vi "The Shell.vi"() -> ()   [LabVIEW 2010]
uses:
  Global variables/Parameters.glb
panel:
  in  "Directory for Saved Data":path=path "D:/Data"
  out "found match":bool
  in  "New session?":bool
  in  "Animal type":u16(ring) items=["Frog", "Gecko", "Chicken", "Probe", "Lamprey"]
  in  "New ear?":bool
  out "Instructions":string="Click once on your name; then select OK.  "
  in  "Stop.":bool
  in  "New cell?":bool
  in  "OK.":bool
  out "Choice":string
  out "Display.":string
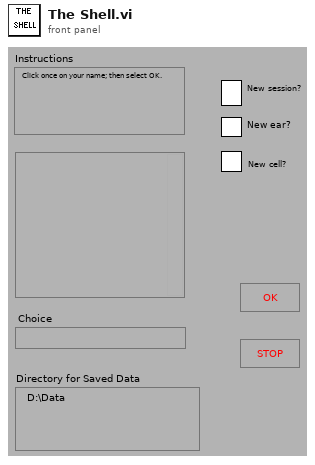
[diagram p1: front panel]
types:
  T1 = enum16{"open", "replace", "create", "open or create", "replace or create", "replace or create with confirmation"}
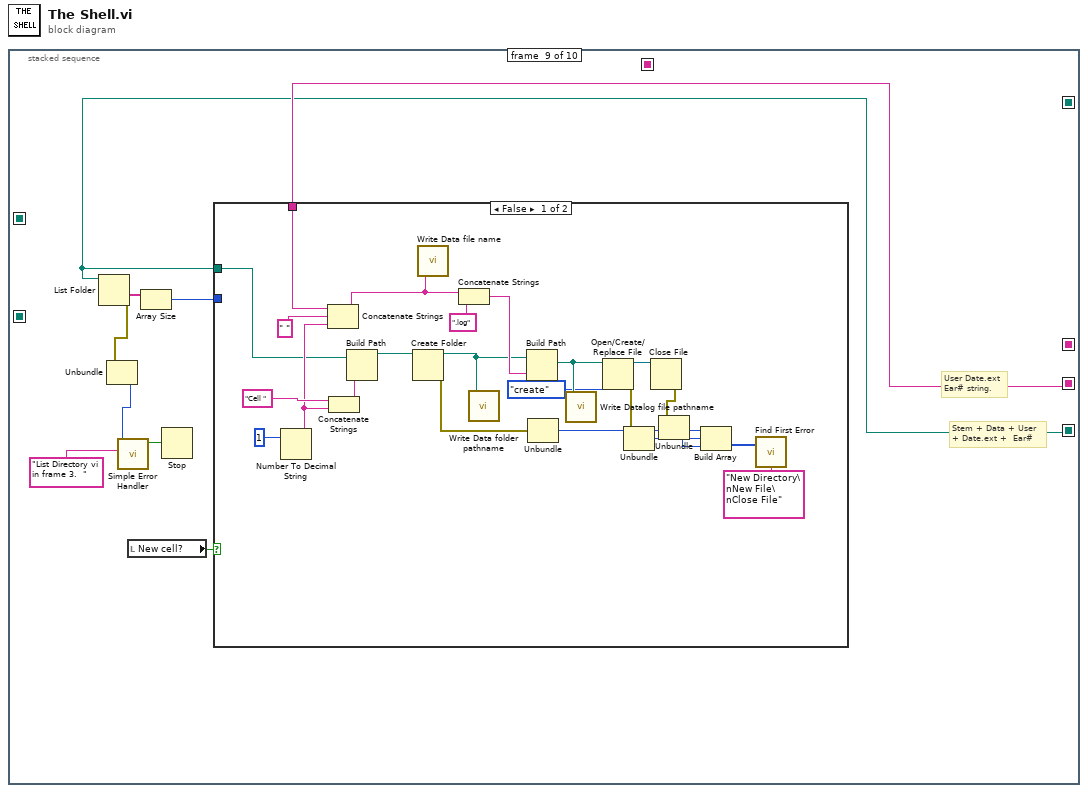
[diagram p0: block diagram]
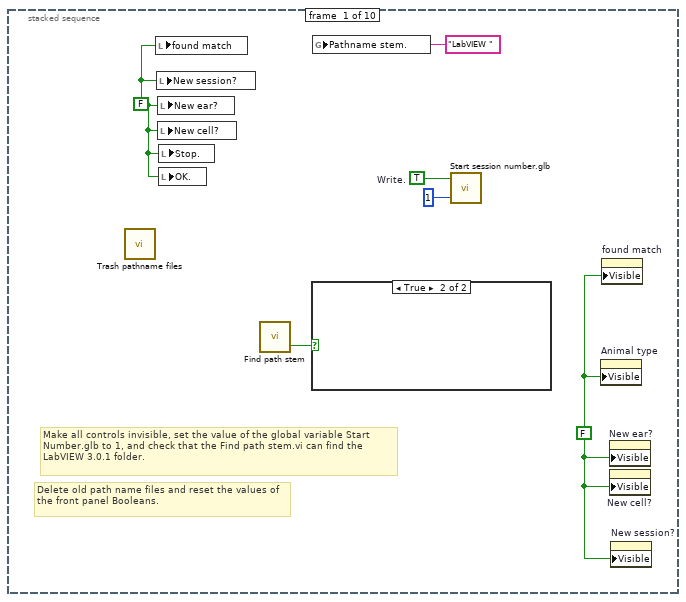
[diagram p2: hidden frame]
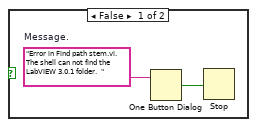
[diagram p3: hidden frame]
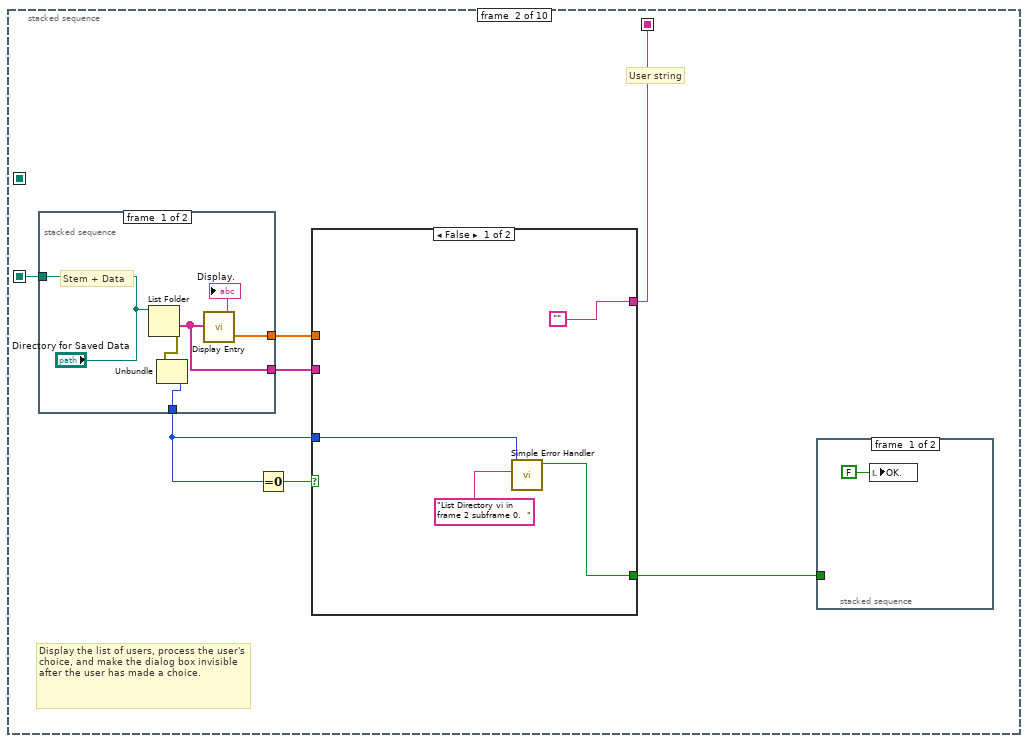
[diagram p4: hidden frame]
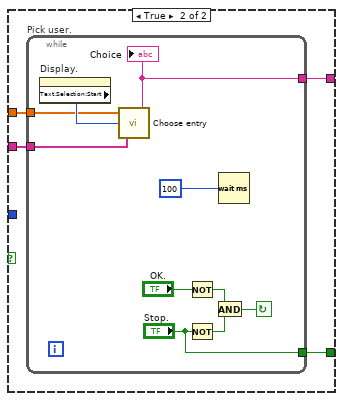
[diagram p5: hidden frame]
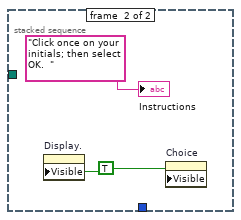
[diagram p6: hidden frame]
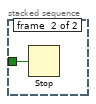
[diagram p7: hidden frame]
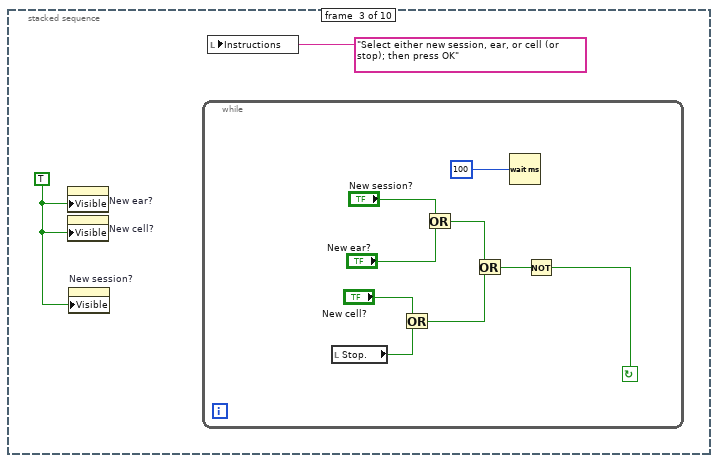
[diagram p8: hidden frame]
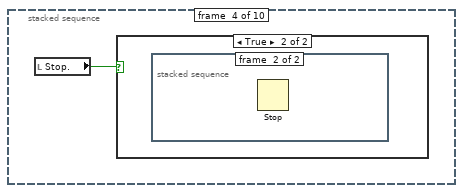
[diagram p9: hidden frame]
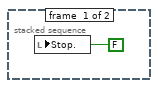
[diagram p11: hidden frame]
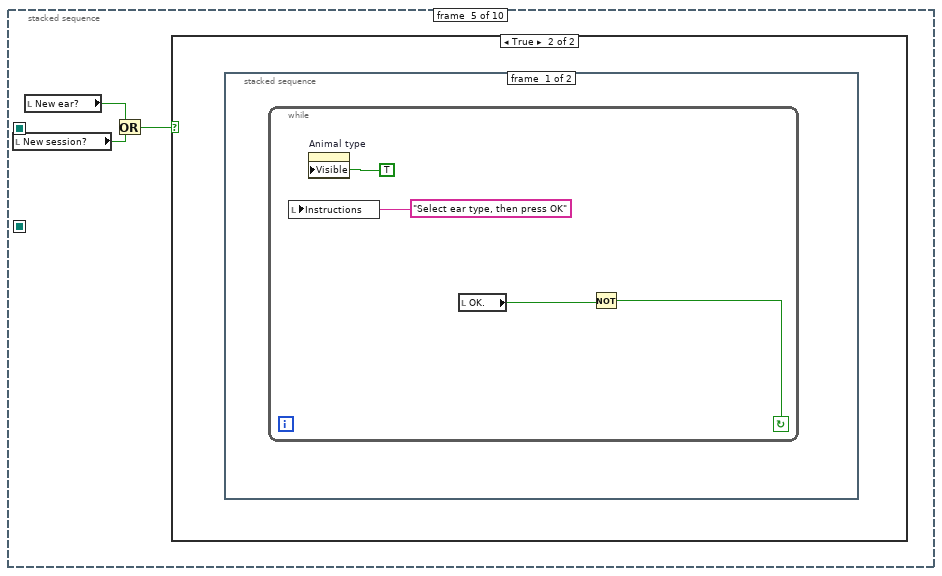
[diagram p12: hidden frame]
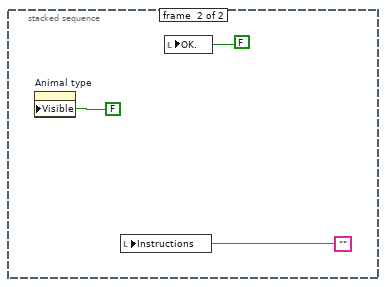
[diagram p14: hidden frame]
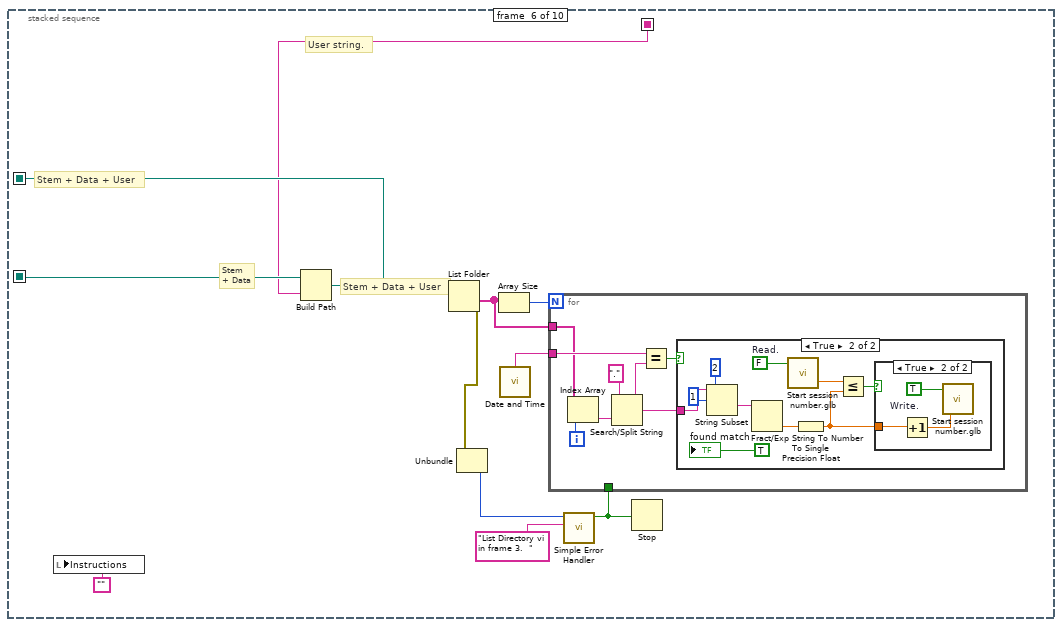
[diagram p15: hidden frame]
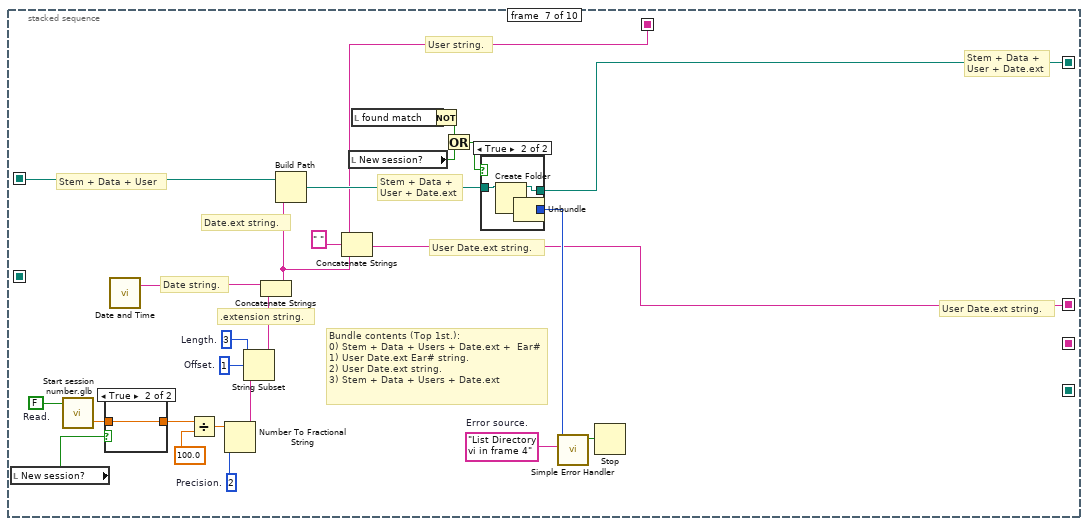
[diagram p18: hidden frame]
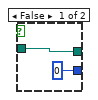
[diagram p19: hidden frame]
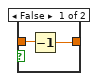
[diagram p20: hidden frame]
diagram:
  n1 = stacked-sequence {
    seq-local: [_ w10 _ _ _ _ _ _ _ _] -> [_ _ _ _ _ w68 w99 _ _ _]
    seq-local: [_ w15 _ _ _ _ _ _ _ _] -> [_ _ _ _ _ w76 _ _ _ _]
    seq-local: [_ _ _ _ _ w69 _ _ _ _] -> [_ _ _ _ _ _ w111 _ _ _]
    seq-local: [_ _ _ _ _ _ w105 _ _ _] -> [_ _ _ _ _ _ _ w137 _ _]
    seq-local: [_ _ _ _ _ _ w104 _ _ _] -> [_ _ _ _ _ _ _ w138 _ _]
    seq-local: [_ _ _ _ _ _ _ w136 _ _] -> [_ _ _ _ _ _ _ _ w189 _]
    seq-local: [_ _ _ _ _ _ _ w135 _ _] -> [_ _ _ _ _ _ _ _ w185 _]
    frame #0 {
      w3 = FALSE
      w2 = FALSE
      w6 = TRUE  # Write.
      # "Delete old path name files and reset the values of the front panel Booleans."
      # "Make all controls invisible, set the value of the global variable Start Number.glb to 1, and check that the Find path stem.vi can find the LabVIEW 3.0.1 folder."
      n2 = call "Trash pathname files.vi"() -> ()  [unwired: 1 in, 2 out]
      n3 = local write "found match"(w2) -> ()
      n4 = local write "New session?"(w2) -> ()
      n5 = local write "New ear?"(w2) -> ()
      n6 = local write "New cell?"(w2) -> ()
      n7 = local write "Stop."(w2) -> ()
      n8 = local write "OK."(w2) -> ()
      n9 = call "Find path stem.vi"() -> ("PASS/FAIL"=w4:bool)  [unwired: 1 out]
      n10 = case shown="True" w4 {
        frame False {
          w7 = "Error in Find path stem.vi.  The shell can not find the LabVIEW 3.0.1 folder.  "  # Message.
          n11 = One Button Dialog(message=w7) -> (true=w8:bool)  [unwired: 1 out]
          n12 = Stop(stop? (T)=w8) -> ()
        }
        frame True {
        }
      }
      n13 = global write "Parameters.glb" "Pathname stem."("LabVIEW ") -> ()
      n14 = call "Start session number.glb"("x."=1, "Mode."=w6) -> ()  [unwired: 2 out]
      n15 = property on="Animal type" class="Ring (strict)"("Visible"=w3) -> ()  [unwired: 2 in, 2 out]
      n16 = property on="found match" class="Bool (strict)"("Visible"=w3) -> ()  [unwired: 2 in, 2 out]
      n17 = property on="New ear?" class="Bool (strict)"("Visible"=w3) -> ()  [unwired: 2 in, 2 out]
      n18 = property on="New cell?" class="Bool (strict)"("Visible"=w3) -> ()  [unwired: 2 in, 2 out]
      n19 = property on="New session?" class="Bool (strict)"("Visible"=w3) -> ()  [unwired: 2 in, 2 out]
    }
    frame #1 {
      # "User string"
      # "Display the list of users, process the user's choice, and make the dialog box invisible after the user has made a choice."
      n20 = stacked-sequence {
        tunnel: [w39 _] -> w13
        tunnel: [w38 _] -> w14
        tunnel: ["Directory for Saved Data" _] -> w15
        tunnel: [w35 _] -> w9
        frame #0 {
          # "Stem + Data"
          n21 = List Folder(path="Directory for Saved Data") -> (folder names=w39:string[], error out=w36:errorcluster)  [unwired: 1 in, 4 out]
          n22 = Unbundle(w36) -> ("code"=w35:i32)  [unwired: 2 out]
          n23 = call "Display Entry.vi"("Array of strings."=w39) -> ("Single string."=→"Display.":string, "Array of string lengths."=w38:sgl[])
        }
        frame #1 {
          w40 = TRUE
          n24 = property on="Display." class="Str"("Visible"=w40) -> ()  [unwired: 2 in, 2 out]
          n25 = property on="Choice" class="Str"("Visible"=w40) -> ()  [unwired: 2 in, 2 out]
          "Instructions" <- "Click once on your initials; then select OK.  "
        }
      }
      n26 = Equal To 0?(x=w9) -> (x = 0?=w11:bool)
      n27 = case shown="False" w11 {
        tunnel: w14 -> [_ w23]
        tunnel: w13 -> [_ w22]
        tunnel: [w16 w21] -> w12
        tunnel: ["" w20] -> w10
        tunnel: w9 -> [w18 _]
        frame False {
          n28 = call <vilib>:"Simple Error Handler.vi"("error code (no error:0)"=w18, "error source (\" \")"="List Directory vi in frame 2 subframe 0.  ") -> ("error?"=w16:bool)  [unwired: 2 in, 5 out]
        }
        frame True {
          n29 = while "Pick user." {
            tunnel: ["Stop."] -> w21
            tunnel: [w25] -> w20
            tunnel: w23 -> [w31]
            tunnel: w22 -> [w32]
            stop <- w28 continue-if-true
            n30 = property on="Display." class="Str"() -> ("Text.Selection:Start"=w33:u32)  [unwired: 2 in, 2 out]
            n31 = call "Choose entry.vi"("Array of strings."=w32, "Selection start."=w33, "Array of string lengths."=w31) -> ("Selected string."=w25:string)
            "Choice" <- w25
            n32 = Not(x="OK.") -> (.not. x?=w29:bool)
            n33 = Not(x="Stop.") -> (.not. x?=w26:bool)
            n34 = And(x=w29, y=w26) -> (x .and. y?=w28:bool)
            n35 = Wait (ms)(milliseconds to wait=100) -> ()  [unwired: 1 out]
          }
        }
      }
      n36 = stacked-sequence {
        tunnel: w12 -> [_ w43]
        frame #0 {
          n37 = local write "OK."(FALSE) -> ()
        }
        frame #1 {
          n38 = Stop(stop? (T)=w43) -> ()
        }
      }
    }
    frame #2 {
      w44 = TRUE
      n39 = property on="New ear?" class="Bool (strict)"("Visible"=w44) -> ()  [unwired: 2 in, 2 out]
      n40 = property on="New cell?" class="Bool (strict)"("Visible"=w44) -> ()  [unwired: 2 in, 2 out]
      n41 = property on="New session?" class="Bool (strict)"("Visible"=w44) -> ()  [unwired: 2 in, 2 out]
      n42 = while {
        stop <- w50 continue-if-true
        n43 = local read "Stop."() -> (w48:bool)
        n44 = Or(x="New cell?", y=w48) -> (x .or. y?=w47:bool)
        n45 = Or(x="New session?", y="New ear?") -> (x .or. y?=w52:bool)
        n46 = Or(x=w52, y=w47) -> (x .or. y?=w51:bool)
        n47 = Wait (ms)(milliseconds to wait=100) -> ()  [unwired: 1 out]
        n48 = Not(x=w51) -> (.not. x?=w50:bool)
      }
      n49 = local write "Instructions"("Select either new session, ear, or cell (or stop); then press OK") -> ()
    }
    frame #3 {
      n50 = local read "Stop."() -> (w55:bool)
      n51 = case shown="True" w55 {
        frame False {
        }
        frame True {
          n52 = stacked-sequence {
            frame #0 {
              n53 = local write "Stop."(FALSE) -> ()
            }
            frame #1 {
              n54 = Stop() -> ()  [unwired: 1 out]
            }
          }
        }
      }
    }
    frame #4 {
      n55 = local read "New session?"() -> (w58:bool)
      n56 = local read "New ear?"() -> (w59:bool)
      n57 = Or(x=w59, y=w58) -> (x .or. y?=w57:bool)
      n58 = case shown="True" w57 {
        frame False {
        }
        frame True {
          n59 = stacked-sequence {
            frame #0 {
              n60 = while {
                stop <- w60 continue-if-true
                n61 = local write "Instructions"("Select ear type, then press OK") -> ()
                n62 = property on="Animal type" class="Ring (strict)"("Visible"=TRUE) -> ()  [unwired: 2 in, 2 out]
                n63 = local read "OK."() -> (w61:bool)
                n64 = Not(x=w61) -> (.not. x?=w60:bool)
              }
            }
            frame #1 {
              n65 = property on="Animal type" class="Ring (strict)"("Visible"=FALSE) -> ()  [unwired: 2 in, 2 out]
              n66 = local write "Instructions"("") -> ()
              n67 = local write "OK."(FALSE) -> ()
            }
          }
        }
      }
    }
    frame #5 {
      # "Stem + Data + User"
      # "User string."
      # "Stem + Data"
      # "Stem + Data + User"
      n68 = local write "Instructions"("") -> ()
      n69 = Build Path(base path=w76, name or relative path=w68) -> (appended path=w69:path)
      n70 = List Folder(path=w69) -> (folder names=w70:string[], error out=w75:errorcluster)  [unwired: 1 in, 4 out]
      n71 = Unbundle(w75) -> ("code"=w67:i32)  [unwired: 2 out]
      n72 = Array Size(array=w70) -> (size(s)=w72:i32)
      n73 = call "Date and Time.vi"() -> ("Date string."=w71:string)  [unwired: 1 out]
      n74 = call <vilib>:"Simple Error Handler.vi"("error code (no error:0)"=w67, "error source (\" \")"="List Directory vi in frame 3.  ") -> ("error?"=w74:bool)  [unwired: 2 in, 5 out]
      n75 = for {
        N: w72 -> [_]
        tunnel: w71 -> [w83]
        tunnel: w74 -> [_]
        tunnel: w70 -> [w78]
        i -> [w85]
        n76 = Index Array(array=w78, index=w85) -> (element=w82:string)
        n77 = Search/Split String(string=w82, search string/char (-)=".") -> (substring before match=w80:string, match + rest of string=w79:string)  [unwired: 2 out]
        n78 = Equal?(x=w83, y=w80) -> (x = y?=w84:bool)
        n79 = case shown="True" w84 {
          tunnel: w79 -> [_ w92]
          frame False {
          }
          frame True {
            w95 = FALSE  # Read.
            n80 = String Subset(string=w92, offset (0)=1, length (rest)=2) -> (substring=w91:string)
            n81 = Fract/Exp String To Number(string=w91) -> (number=w88:dbl)  [unwired: 4 out]
            n82 = call "Start session number.glb"("Mode."=w95) -> ("x."=w89:sgl)  [unwired: 1 in, 1 out]
            n83 = To Single Precision Float(number=w88) -> (single precision float=w86:sgl)
            n84 = Less Or Equal?(x=w89, y=w86) -> (x <= y?=w90:bool)
            n85 = case shown="True" w90 {
              tunnel: w86 -> [_ w97]
              frame False {
              }
              frame True {
                w98 = TRUE  # Write.
                n86 = Increment(x=w97) -> (x+1=w96:sgl)
                n87 = call "Start session number.glb"("x."=w96, "Mode."=w98) -> ()  [unwired: 2 out]
              }
            }
            "found match" <- TRUE
          }
        }
      }
      n88 = Stop(stop? (T)=w74) -> ()
    }
    frame #6 {
      w112 = "List Directory vi in frame 4"  # Error source.
      w118 = 1  # Offset.
      w119 = 3  # Length.
      w120 = 2  # Precision.
      w124 = FALSE  # Read.
      # "User Date.ext string."
      # "Stem + Data + User + Date.ext"
      # "Bundle contents (Top 1st.):  \n0) Stem + Data + Users + Date.ext +  Ear# \n1) User Date.ext Ear# string.  \n2) User Date.ext string.     \n3) Stem + Data + Users + Date.ext"
      # "User Date.ext string."
      # "Stem + Data + User + Date.ext"
      # ".extension string."
      # "Date.ext string."
      # "Date string."
      # "User string."
      # "Stem + Data + User"
      n89 = local read "New session?"() -> (w110:bool)
      n90 = call "Start session number.glb"("Mode."=w124) -> ("x."=w109:sgl)  [unwired: 1 in, 1 out]
      n91 = case shown="True" w110 {
        tunnel: [w131 w133] -> w108
        tunnel: w109 -> [w132 w133]
        frame False {
          n92 = Decrement(x=w132) -> (x-1=w131:sgl)
        }
        frame True {
        }
      }
      n93 = call "Date and Time.vi"() -> ("Date string."=w114:string)  [unwired: 1 out]
      n94 = Divide(x=w108, y=sgl 100.0) -> (x/y=w121:sgl)
      n95 = Number To Fractional String(number=w121, precision (6)=w120) -> (F-format string=w117:string)  [unwired: 2 out]
      n96 = String Subset(string=w117, offset (0)=w118, length (rest)=w119) -> (substring=w116:string)
      n97 = Concatenate Strings(w114, w116) -> (w115:string)
      n98 = Build Path(base path=w111, name or relative path=w115) -> (appended path=w107:path)
      n99 = Concatenate Strings(w99, " ", w115) -> (w104:string)
      n100 = local read "New session?"() -> (w101:bool)
      n101 = local read "found match"() -> (w103:bool)
      n102 = Not(x=w103) -> (.not. x?=w102:bool)
      n103 = Or(x=w102, y=w101) -> (x .or. y?=w100:bool)
      n104 = case shown="True" w100 {
        tunnel: [w126 w129] -> w105
        tunnel: w107 -> [w126 w130]
        tunnel: [0 w127] -> w106
        frame False {
        }
        frame True {
          n105 = Create Folder(path (use dialog)=w130) -> (created path=w129:path, error out=w128:errorcluster)  [unwired: 1 in, 2 out]
          n106 = Unbundle(w128) -> ("code"=w127:i32)  [unwired: 2 out]
        }
      }
      n107 = call <vilib>:"Simple Error Handler.vi"("error code (no error:0)"=w106, "error source (\" \")"=w112) -> ("error?"=w113:bool)  [unwired: 2 in, 5 out]
      n108 = Stop(stop? (T)=w113) -> ()
    }
    frame #7 {
      # "Stem + Data + User + Date.ext"
      n109 = List Folder(path=w137) -> (folder names=w141:string[], error out=w144:errorcluster)  [unwired: 1 in, 4 out]
      n110 = Unbundle(w144) -> ("code"=w134:i32)  [unwired: 2 out]
      n111 = call <vilib>:"Simple Error Handler.vi"("error code (no error:0)"=w134, "error source (\" \")"="List Directory vi in frame 3.  ") -> ("error?"=w142:bool)  [unwired: 2 in, 5 out]
      n112 = local read "New ear?"() -> (w140:bool)
      n113 = Array Size(array=w141) -> (size(s)=w139:i32)
      n114 = Stop(stop? (T)=w142) -> ()
      n115 = case shown="False" w140 {
        tunnel: w139 -> [w149 w171]
        tunnel: w138 -> [w147 w176]
        tunnel: w137 -> [w148 w174]
        tunnel: [w146 w175] -> w136
        tunnel: [w145 w173] -> w135
        frame False {
          n116 = local read "New session?"() -> (w150:bool)
          n117 = case shown="True" w150 {
            tunnel: w149 -> [w153 _]
            tunnel: w148 -> [w152 w164]
            tunnel: w147 -> [w151 w165]
            tunnel: [w155 w162] -> w146
            tunnel: [w154 w161] -> w145
            frame False {
              n118 = Number To Decimal String(number=w153) -> (decimal integer string=w156:string)  [unwired: 1 out]
              n119 = Concatenate Strings(w151, " ", w156) -> (w155:string)
              n120 = Concatenate Strings("Ear ", w156) -> (w159:string)
              n121 = Build Path(base path=w152, name or relative path=w159) -> (appended path=w154:path)
            }
            frame True {
              # "Error bundle."
              n122 = call "Make ear folder.vi"("Ear folder number."=1, "Date folder path name."=w164, "Date folder path name (string)."=w165) -> ("Error bundle out."=w166:errorcluster, "Ear folder path name."=w161:path, "Ear folder path name (string)."=w162:string)  [unwired: 1 in]
              n123 = call <vilib>:"Simple Error Handler.vi"("error in (no error)"=w166) -> ("error?"=w167:bool)  [unwired: 1 in, 7 out]
              n124 = local read "Animal type"() -> (w160:u16)
              n125 = Stop(stop? (T)=w167) -> ()
              n126 = case shown="..0" w160 {
                tunnel: w161 -> [w168 w169 _ _]
                frame ..0 {
                  n127 = call "Frog ear specs.vi"("ear folder path"=w168) -> ()
                }
                frame 1 {
                  n128 = call "Gecko anesthesia specs.vi"("ear folder path"=w169) -> ()
                }
                frame 2 {
                }
                frame 3.. {
                }
              }
            }
          }
        }
        frame True {
          # "Error bundle."
          n129 = Increment(x=w171) -> (x+1=w170:i32)
          n130 = call "Make ear folder.vi"("Ear folder number."=w170, "Date folder path name."=w174, "Date folder path name (string)."=w176) -> ("Error bundle out."=w177:errorcluster, "Ear folder path name."=w173:path, "Ear folder path name (string)."=w175:string)  [unwired: 1 in]
          n131 = call <vilib>:"Simple Error Handler.vi"("error in (no error)"=w177) -> ("error?"=w178:bool)  [unwired: 1 in, 7 out]
          n132 = Stop(stop? (T)=w178) -> ()
          n133 = case shown="..0" "Animal type" {
            tunnel: w173 -> [w179 w180 _ _]
            frame ..0 {
              n134 = call "Frog ear specs.vi"("ear folder path"=w179) -> ()
            }
            frame 1 {
              n135 = call "Gecko anesthesia specs.vi"("ear folder path"=w180) -> ()
            }
            frame 2 {
            }
            frame 3.. {
            }
          }
        }
      }
    }
    frame #8 {
      # "Stem + Data + User + Date.ext +  Ear#"
      # "User Date.ext Ear# string."
      n136 = List Folder(path=w185) -> (folder names=w186:string[], error out=w187:errorcluster)  [unwired: 1 in, 4 out]
      n137 = Unbundle(w187) -> ("code"=w181:i32)  [unwired: 2 out]
      n138 = call <vilib>:"Simple Error Handler.vi"("error code (no error:0)"=w181, "error source (\" \")"="List Directory vi in frame 3.  ") -> ("error?"=w183:bool)  [unwired: 2 in, 5 out]
      n139 = local read "New cell?"() -> (w188:bool)
      n140 = Array Size(array=w186) -> (size(s)=w182:i32)
      n141 = Stop(stop? (T)=w183) -> ()
      n142 = case shown="False" w188 {
        tunnel: w189 -> [w196 w217]
        tunnel: w185 -> [w195 w216]
        tunnel: w182 -> [_ w214]
        frame False {
          n143 = Number To Decimal String(number=1) -> (decimal integer string=w208:string)  [unwired: 1 out]
          n144 = Concatenate Strings(w196, " ", w208) -> (w203:string)
          n145 = Concatenate Strings("Cell ", w208) -> (w211:string)
          n146 = Build Path(base path=w195, name or relative path=w211) -> (appended path=w212:path)
          n147 = Create Folder(path (use dialog)=w212) -> (created path=w204:path, error out=w202:errorcluster)  [unwired: 1 in, 2 out]
          n148 = call "Write Data file name.vi"("Data file name."=w203) -> ()  [unwired: 1 out]
          n149 = Concatenate Strings(w203, ".log") -> (w206:string)
          n150 = call "Write Data folder pathname.vi"("Data folder pathname."=w204) -> ()  [unwired: 1 out]
          n151 = Build Path(base path=w204, name or relative path=w206) -> (appended path=w194:path)
          n152 = Unbundle(w202) -> ("code"=w191:i32)  [unwired: 2 out]
          n153 = call "Write Datalog file pathname.vi"("Datalog file pathname."=w194) -> ()  [unwired: 1 out]
          n154 = Open/Create/Replace File(file path (use dialog)=w194, operation (0:open)=T1."create") -> (refnum out=w205:refnum<file>, error out=w201:errorcluster)  [unwired: 1 in, 4 out]
          n155 = Unbundle(w201) -> ("code"=w192:i32)  [unwired: 2 out]
          n156 = Close File(refnum=w205) -> (error out=w200:errorcluster)  [unwired: 1 in, 1 out]
          n157 = Unbundle(w200) -> ("code"=w193:i32)  [unwired: 2 out]
          n158 = Build Array(w191, w192, w193) -> (w199:i32[])
          n159 = call <vilib>:"Find First Error.vi"("source messages"="New Directory\nNew File\nClose File", "error codes"=w199) -> ()  [unwired: 1 in, 3 out]
        }
        frame True {
          # "Error bundle."
          n160 = Increment(x=w214) -> (x+1=w215:i32)
          n161 = call "Make cell folder.vi"("Cell folder number."=w215, "Ear folder path name."=w216, "Ear folder path name (string)."=w217) -> ("Error bundle out."=w218:errorcluster)  [unwired: 1 in]
          n162 = call <vilib>:"Simple Error Handler.vi"("error in (no error)"=w218) -> ("error?"=w213:bool)  [unwired: 1 in, 7 out]
          n163 = Stop(stop? (T)=w213) -> ()
        }
      }
    }
    frame #9 {
      w219 = FALSE
      n164 = local write "New session?"(w219) -> ()
      n165 = local write "New cell?"(w219) -> ()
      n166 = local write "New ear?"(w219) -> ()
      n167 = local write "Stop."(w219) -> ()
      n168 = local write "OK."(w219) -> ()
    }
  }
